vi "dfd_FXPSimu AccSub (scaler).vi"(5 "quantize output?":bool, 7 "FXP OP":T4={"source"=0, "is floating?"=FALSE, "o-mode"=enum."Wrap", "q-mode"=enum."Nearest", "signed?"=FALSE, "fwl"=0, "high limit"=0.0, "low limit"=0.0, "full range"=0.0} {"source" items=["Coef a/k"=0, "Coef b/v"=7, "Input"=1, "Output"=2, "Multiplicand"=3, "Product"=4, "Sum"=5, "Delay"=6, "Gain"=8]}, 8 "filtering statistics in":T3(array[cluster]) {"statistics information"."min value" format="%.2f"; "statistics information"."max value" format="%.2f"; "Quantizer Source" items=["Coefficients a/k"=0, "Coefficients b/v"=7, "Input"=1, "Output"=2, "Multiplicand"=3, "Product"=4, "Sum"=5, "Delay"=6]}, 10 "addend":ext format="%.2f", 11 "acc in":ext format="%.2f") -> (0 "filtering statistics out":T3(array[cluster]) {"statistics information"."min value" format="%.2f"; "statistics information"."max value" format="%.2f"; "Quantizer Source" items=["Coefficients a/k"=0, "Coefficients b/v"=7, "Input"=1, "Output"=2, "Multiplicand"=3, "Product"=4, "Sum"=5, "Delay"=6]}, 3 "acc out":ext format="%.2f")   [LabVIEW 2017, in "NI_DigFilter_FXP.lvlib"]
uses:
  <vilib>/addons/Digital Filter Design/NI_DigFilter_FXP.lvlib
  <vilib>/addons/Digital Filter Design/_Objects.llb/dfd_FXP Operation.ctl
  <vilib>/addons/Digital Filter Design/_Objects.llb/dfd_Internal Quantization Srcs.ctl
  <vilib>/addons/Digital Filter Design/_Objects.llb/DFD Quantization Sources.ctl
  <vilib>/addons/Digital Filter Design/_Objects.llb/DFD FXP Statistics Data.ctl
  <vilib>/addons/Digital Filter Design/NI_DigFilterLicensed.lvlib
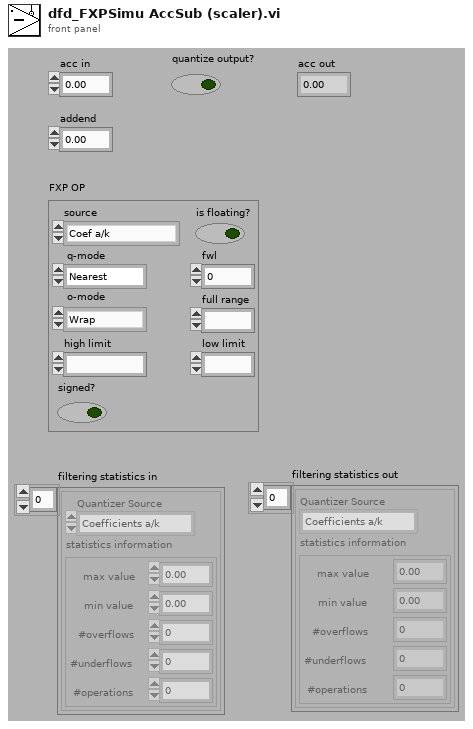
[diagram p1: front panel]
types:
  T1 = typedef "NI_DigFilterLicensed.lvlib/DFD Quantization Sources.ctl" = u16
  T2 = typedef "NI_DigFilterLicensed.lvlib/DFD FXP Statistics Data.ctl" = cluster{"max value":ext, "min value":ext, "#overflows":i32, "#underflows":i32, "#operations":i32}
  T3 = cluster{"Quantizer Source":T1, "statistics information":T2}[]
  T4 = typedef "dfd_FXP Operation.ctl" = cluster{"source":T5, "is floating?":bool, "o-mode":enum16{"Saturation", "Wrap"}, "q-mode":enum16{"Nearest", "Truncation"}, "signed?":bool, "fwl":i16, "high limit":ext, "low limit":ext, "full range":ext}
  T5 = typedef "NI_DigFilterLicensed.lvlib/dfd_Internal Quantization Srcs.ctl" = u16
  T6 = cluster{"Quantizer Source":T1, "statistics information":T2}
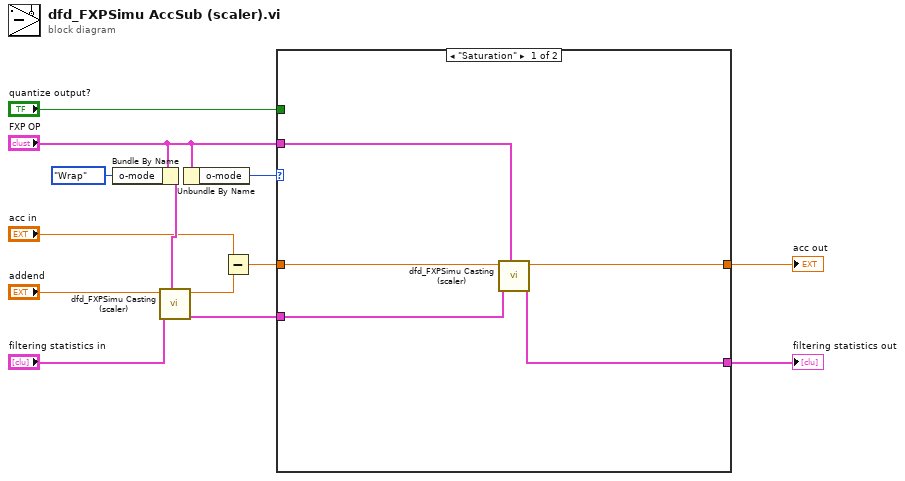
[diagram p0: block diagram]
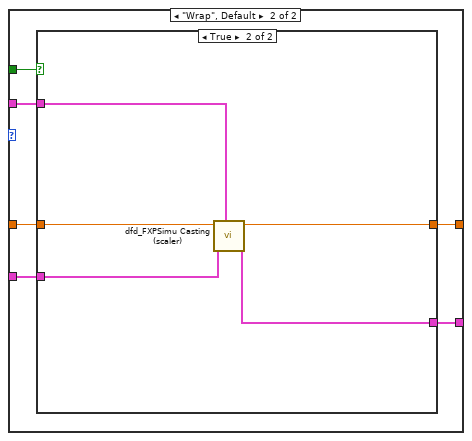
[diagram p2: hidden frame]
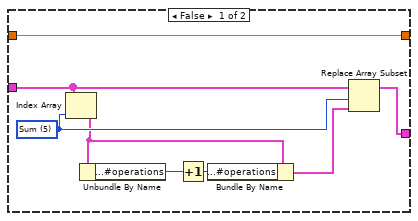
[diagram p3: hidden frame]
diagram:
  n1 = Bundle By Name(cluster="FXP OP", "o-mode"=enum16{"Saturation", "Wrap"}."Wrap" ("o_mode")) -> (w7:T4)
  n2 = call <vilib>:"dfd_FXPSimu Casting (scaler).vi"("FXP op"=w7, "filtering statistics in"="filtering statistics in", "value in"="addend") -> ("filtering statistics out"=w6:T3, "value out"=w10:ext)  [unwired: 7 out]
  n3 = Unbundle By Name("FXP OP") -> ("o-mode"=w3:enum16{"Saturation", "Wrap"})
  n4 = Subtract(x="acc in", y=w10) -> (x-y=w13:ext)
  n5 = case shown="\"Saturation\"" w3 {
    tunnel: w13 -> [w18 w23]
    tunnel: [w17 w21] -> w12
    tunnel: [w14 w19] -> w9
    tunnel: w6 -> [w16 w20]
    tunnel: "quantize output?" -> [_ w24]
    tunnel: "FXP OP" -> [w15 w22]
    frame "Saturation" {
      n6 = call <vilib>:"dfd_FXPSimu Casting (scaler).vi"("FXP op"=w15, "filtering statistics in"=w16, "value in"=w18) -> ("filtering statistics out"=w14:T3, "value out"=w17:ext)  [unwired: 7 out]
    }
    frame "Wrap", Default {
      n7 = case shown="True" w24 {
        tunnel: w23 -> [w32 w37]
        tunnel: w22 -> [_ w36]
        tunnel: [w32 w35] -> w21
        tunnel: w20 -> [w31 w34]
        tunnel: [w30 w33] -> w19
        frame False {
          w29 = T5 5 items=["Coef a/k"=0, "Coef b/v"=7, "Input"=1, "Output"=2, "Multiplicand"=3, "Product"=4, "Sum"=5, "Delay"=6, "Gain"=8] ("source")
          n8 = Index Array(array=w31, index=w29) -> (element=w28:T6)
          n9 = Unbundle By Name(w28) -> ("statistics information.#operations"=w27:i32)
          n10 = Increment(x=w27) -> (x+1=w26:i32)
          n11 = Bundle By Name(cluster=w28, "statistics information.#operations"=w26) -> (w25:T6)
          n12 = Replace Array Subset(array=w31, new element=w25, index=w29) -> (w30:T3)
        }
        frame True {
          n13 = call <vilib>:"dfd_FXPSimu Casting (scaler).vi"("FXP op"=w36, "filtering statistics in"=w34, "value in"=w37) -> ("filtering statistics out"=w33:T3, "value out"=w35:ext)  [unwired: 7 out]
        }
      }
    }
  }
  "acc out" <- w12
  "filtering statistics out" <- w9
